vi "Write Cluster.vi"(8 "error in":errorcluster, 9 "Cluster":variant, 10 "Group Name":string, 11 "tdms file in":refnum<k34>) -> (0 "error out":errorcluster, 2 "Group Name":string, 3 "tdms file out":refnum<k34>)   [LabVIEW 2010]
panel:
  # "Writes the given cluster\nto the given TDMS file."
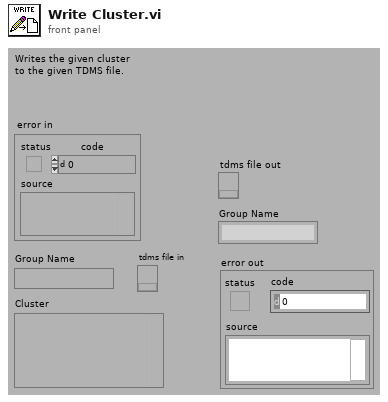
[diagram p1: front panel]
types:
  T1 = typedef "Type Descriptor Enumeration__ogtk.ctl" = enum8{"<Null>", "I8", "I16", "I32", "I64", "U8", "U16", "U32", "U64", "SGL", "DBL", "EXT", "CSG", "CDB", "CXT", "0x0F", "0x10", "0x11", "0x12", "0x13", "0x14", "Enum U8", "Enum U16", "Enum U32", "Enum U64", "SGL PQ", "DBL PQ", "EXT PQ", "CSG PQ", "CDB PQ", "CXT PQ", "0x1F", "0x20", "Boolean", "0x22", "0x23", "0x24", "0x25", "0x26", "0x27", "0x28", "0x29", "0x2A", "0x2B", "0x2C", "0x2D", "0x2E", "0x2F", "String", "0x31", "Path", "Pict", "0x34", "0x35", "0x36", "DAQ", "0x38", "0x39", "0x3A", "0x3B", "0x3C", "0x3D", "0x3E", "0x3F", "Array", "0x41", "0x42", "0x43", "0x44", "0x45", "0x46", "0x47", "0x48", "0x49", "0x4A", "0x4B", "0x4C", "0x4D", "0x4E", "0x4F", "Cluster", "0x51", "0x52", "Variant", "Waveform", "0x55", "0x56", "0x57", "0x58", "0x59", "0x5A", "0x5B", "0x5C", "0x5D", "0x5E", "0x5F", "0x60", "0x61", "0x62", "0x63", "0x64", "0x65", "0x66", "0x67", "0x68", "0x69", "0x6A", "0x6B", "0x6C", "0x6D", "0x6E", "0x6F", "Refnum"}
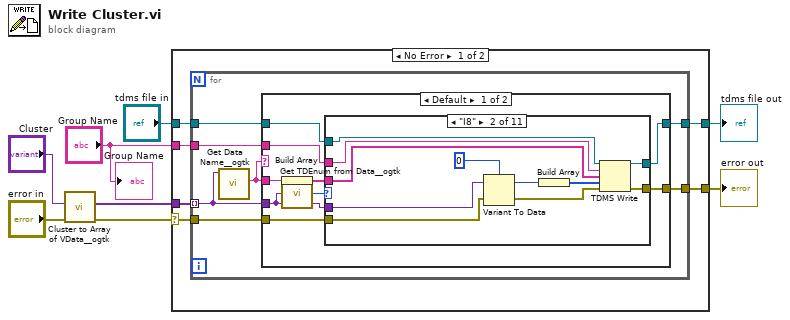
[diagram p0: block diagram]
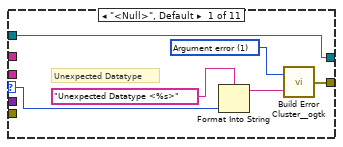
[diagram p2: hidden frame]
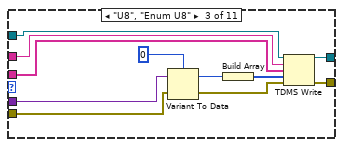
[diagram p3: hidden frame]
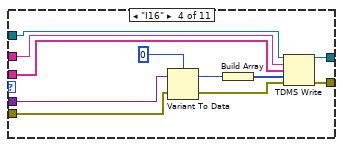
[diagram p4: hidden frame]
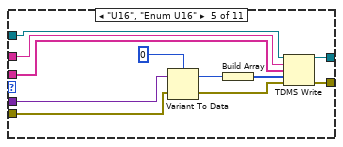
[diagram p5: hidden frame]
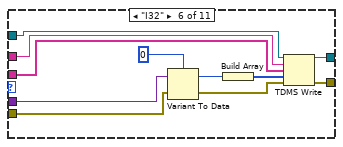
[diagram p6: hidden frame]
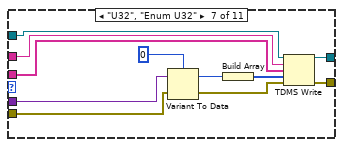
[diagram p7: hidden frame]
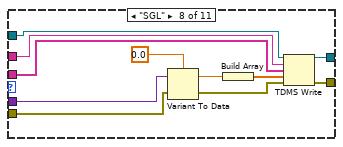
[diagram p8: hidden frame]
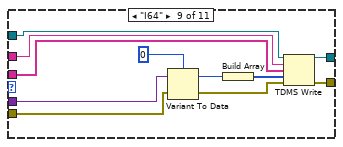
[diagram p9: hidden frame]
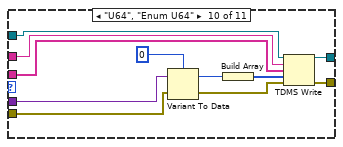
[diagram p10: hidden frame]
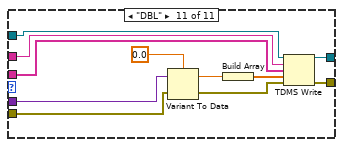
[diagram p11: hidden frame]
diagram:
  n1 = call <userlib>:"Cluster to Array of VData__ogtk.vi"("error in (no error)"="error in", "Cluster"="Cluster") -> ("error out"=w4:errorcluster, "Array of VData"=w8:variant[])  [unwired: 8 in]
  n2 = case shown="No Error" w4 {
    selector: w4 -> [w11 w150]
    tunnel: [w10 w150] -> w5
    tunnel: w8 -> [w12 _]
    tunnel: "Group Name" -> [w13 _]
    tunnel: "tdms file in" -> [w14 w149]
    tunnel: [w9 w149] -> w6
    frame No Error {
      n3 = for {
        tunnel: w12 -> [w20] mode=indexing
        tunnel: w14 -> [w19]
        tunnel: w13 -> [w18]
        tunnel: w11 -> [w17]
        tunnel: [w16] -> w10
        tunnel: [w15] -> w9
        n4 = call <userlib>:"Get Data Name__ogtk.vi"("Data"=w20) -> ("Data Name"=w21:string)  [unwired: 8 in, 2 out]
        n5 = case shown="Default" w21 {
          tunnel: w21 -> [w26 _]
          tunnel: w20 -> [w27 _]
          tunnel: w19 -> [w29 w147]
          tunnel: w18 -> [w24 _]
          tunnel: w17 -> [w30 w148]
          tunnel: [w22 w148] -> w16
          tunnel: [w23 w147] -> w15
          frame Default {
            n6 = Build Array(w26) -> (w25:string[])
            n7 = call <userlib>:"Get TDEnum from Data__ogtk.vi"("Data"=w27) -> ("Type Descriptor Enumeration"=w28:T1)  [unwired: 4 in]
            n8 = case shown="\"I8\"" w28 {
              selector: w28 -> [w33 _ _ _ _ _ _ _ _ _ _]
              tunnel: w30 -> [_ w46 w54 w67 w78 w89 w101 w110 w122 w133 w144]
              tunnel: [w31 w43 w52 w65 w76 w87 w99 w111 w120 w131 w142] -> w22
              tunnel: w29 -> [w32 w39 w57 w63 w73 w84 w94 w106 w117 w128 w139]
              tunnel: w27 -> [_ w45 w51 w68 w79 w90 w97 w109 w123 w134 w145]
              tunnel: [w32 w40 w48 w64 w72 w81 w98 w103 w114 w125 w136] -> w23
              tunnel: w25 -> [_ w42 w55 w59 w70 w82 w92 w104 w115 w126 w137]
              tunnel: w24 -> [_ w41 w56 w60 w71 w83 w93 w105 w116 w127 w138]
              frame "<Null>", Default {
                w34 = 1 items=["No error", "Argument error", "Memory is full", "Out of zone", "End of file", "File already open", "Generic file I/O error", "File not found", "File permission error", "Disk is full", "Duplicate path", "Too many files open", "System feature not enabled", "Resource file not found", "Cannot add resource", "Resource not found", "Image not found", "Image memory error", "Pen does not exist", "Config type invalid", "Config token not found", "Config parse error", "Config memory error", "Bad external code format", "Bad external code offset", "External code not present", "Null window", "Destroy window error", "Null menu", "Print aborted", "Bad print record", "Print driver error", "Windows error during printing", "Memory error during printing", "Print dialog error", "Generic print error", "Invalid device refnum", "Device not found", "Device parameter error", "Device unit error", "Cannot open device", "Device call aborted", "Generic error", "Cancelled by user", "Object ID too low", "Object ID too high", "Object not in heap", "Unknown heap", "Unknown object (invalid DefProc)", "Unknown object (DefProc not in table)", "Message out of range", "Invalid (null) method", "Unknown message", "Manager call not supported", "Bad address", "Network operation in progress", "Network operation timed out", "Connection is busy", "Network attribute not supported", "Network error", "Address in use", "System out of memory", "Connection aborted", "Connection refused", "Not connected", "Already connected", "Connection closed", "Initialization error (interapplication manager)", "Bad occurrence", "Wait on unbound occurrence handler", "Occurrence queue overflow", "Datalog type conflict", "Unused", "Unrecognized type (interapplication manager)", "Memory corrupt", "Failed to make temporary DLL", "Old CIN version", "Drag socket not found", "Failed to load drop-object", "Failed to register OLE object", "Failed to release OLE object", "Format specifier type mismatch", "Unknown format specifier", "Too few format specifiers", "Too many format specifiers", "Scan failed", "Newer CIN version", "Error converting to variant", "Runtime menu error", "Password tampered", "Variant attribute not found", "Incompatible variant data type", "Event data is not available", "Event Store is not present", "Occurrence is not found", "Event Queue is not created", "Event info is not available", "Refnum passed is NULL", "Error retrieving Class GUID", "Error retrieving CoClass GUID", "Error retrieving TypeLib GUID.", "Bad built application magic bytes.", "Specific driver is different from the specific driver associated with the Logical Name.", "There is no session opened to the class driver.", "Max Error", "MAX - Error with config objects", "MAX - Error loading configuration", "MAX - Group not supported"]
                # "Unexpected Datatype"
                n9 = Format Into String(format string="Unexpected Datatype <%s>" ("Format String"), w33) -> (resulting string=w36:string)  [unwired: 2 in, 1 out]
                n10 = call <userlib>:"Build Error Cluster__ogtk.vi"("String to Prepend to source (\"\")"=w36, "code"=w34) -> ("error out"=w31:errorcluster)
              }
              frame "I8" {
                n11 = Variant To Data(error in=w46, Variant=w45, type=i8 0) -> (error out=w44:errorcluster, data=w38:i8)
                n12 = Build Array(w38) -> (w37:i8[])
                n13 = TDMS Write(0:w39, 5:w41, 7:w42, 9:w37, 11:w44) -> (4:w40:refnum<k34>, 15:w43:errorcluster)  [unwired: 1 in, 2 out]
              }
              frame "U8", "Enum U8" {
                n14 = Variant To Data(error in=w54, Variant=w51, type=u8 0) -> (error out=w53:errorcluster, data=w50:u8)
                n15 = Build Array(w50) -> (w49:u8[])
                n16 = TDMS Write(0:w57, 5:w56, 7:w55, 9:w49, 11:w53) -> (4:w48:refnum<k34>, 15:w52:errorcluster)  [unwired: 1 in, 2 out]
              }
              frame "I16" {
                n17 = Variant To Data(error in=w67, Variant=w68, type=i16 0) -> (error out=w66:errorcluster, data=w62:i16)
                n18 = Build Array(w62) -> (w61:i16[])
                n19 = TDMS Write(0:w63, 5:w60, 7:w59, 9:w61, 11:w66) -> (4:w64:refnum<k34>, 15:w65:errorcluster)  [unwired: 1 in, 2 out]
              }
              frame "U16", "Enum U16" {
                n20 = Variant To Data(error in=w78, Variant=w79, type=u16 0) -> (error out=w77:errorcluster, data=w75:u16)
                n21 = Build Array(w75) -> (w74:u16[])
                n22 = TDMS Write(0:w73, 5:w71, 7:w70, 9:w74, 11:w77) -> (4:w72:refnum<k34>, 15:w76:errorcluster)  [unwired: 1 in, 2 out]
              }
              frame "I32" {
                n23 = Variant To Data(error in=w89, Variant=w90, type=0) -> (error out=w88:errorcluster, data=w86:i32)
                n24 = Build Array(w86) -> (w85:i32[])
                n25 = TDMS Write(0:w84, 5:w83, 7:w82, 9:w85, 11:w88) -> (4:w81:refnum<k34>, 15:w87:errorcluster)  [unwired: 1 in, 2 out]
              }
              frame "U32", "Enum U32" {
                n26 = Variant To Data(error in=w101, Variant=w97, type=u32 0) -> (error out=w100:errorcluster, data=w96:u32)
                n27 = Build Array(w96) -> (w95:u32[])
                n28 = TDMS Write(0:w94, 5:w93, 7:w92, 9:w95, 11:w100) -> (4:w98:refnum<k34>, 15:w99:errorcluster)  [unwired: 1 in, 2 out]
              }
              frame "SGL" {
                n29 = Variant To Data(error in=w110, Variant=w109, type=sgl 0.0) -> (error out=w112:errorcluster, data=w108:sgl)
                n30 = Build Array(w108) -> (w107:sgl[])
                n31 = TDMS Write(0:w106, 5:w105, 7:w104, 9:w107, 11:w112) -> (4:w103:refnum<k34>, 15:w111:errorcluster)  [unwired: 1 in, 2 out]
              }
              frame "I64" {
                n32 = Variant To Data(error in=w122, Variant=w123, type=i64 0) -> (error out=w121:errorcluster, data=w119:i64)
                n33 = Build Array(w119) -> (w118:i64[])
                n34 = TDMS Write(0:w117, 5:w116, 7:w115, 9:w118, 11:w121) -> (4:w114:refnum<k34>, 15:w120:errorcluster)  [unwired: 1 in, 2 out]
              }
              frame "U64", "Enum U64" {
                n35 = Variant To Data(error in=w133, Variant=w134, type=u64 0) -> (error out=w132:errorcluster, data=w130:u64)
                n36 = Build Array(w130) -> (w129:u64[])
                n37 = TDMS Write(0:w128, 5:w127, 7:w126, 9:w129, 11:w132) -> (4:w125:refnum<k34>, 15:w131:errorcluster)  [unwired: 1 in, 2 out]
              }
              frame "DBL" {
                n38 = Variant To Data(error in=w144, Variant=w145, type=0.0) -> (error out=w143:errorcluster, data=w141:dbl)
                n39 = Build Array(w141) -> (w140:dbl[])
                n40 = TDMS Write(0:w139, 5:w138, 7:w137, 9:w140, 11:w143) -> (4:w136:refnum<k34>, 15:w142:errorcluster)  [unwired: 1 in, 2 out]
              }
            }
          }
          frame "@dummy control@" {
          }
        }
      }
    }
    frame Error {
    }
  }
  "tdms file out" <- w6
  "error out" <- w5
  "Group Name" <- "Group Name"
